vi "界限转换.vi"() -> ()   [LabVIEW 2018]
panel:
  out "是否强制转换":bool
  out "转化结果":dbl
  in  "数值":dbl
  in  "下限":dbl
  in  "上限":dbl
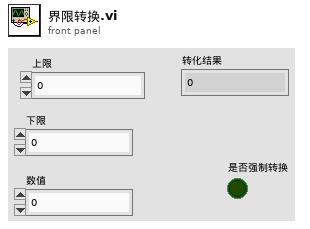
[diagram p1: front panel]
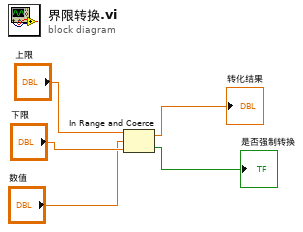
[diagram p0: block diagram]
diagram:
  n1 = In Range and Coerce(upper limit="上限", x="数值", lower limit="下限") -> (coerced(x)=→"转化结果":dbl, In Range?=→"是否强制转换":bool)
